vi "Start Streaming.vi"(8 "error in (no error)":errorcluster, 9 "Camera Settings":T1={"Exposure Time (ms)"=100.0, "Binning"=enum."2x2", "Scan Mode"=-1, "Frames to Acquire"=1000.0, "Pixel Correction"=FALSE, "Frames to Skip"=1, "File Path"=path "", "Duty cycle"=1.0, "ALEX"=FALSE, "Shutter Enable"=[], "fluidics trigger frame"=0, "Bit Depth"=16, "Image Width (px)"=0, "Image Height (px)"=0, "Horizontal Offset (px)"=0, "Vertical Offset (px)"=0} {"fluidics trigger frame" max=60000 step=1; "Exposure Time (ms)" min=1.0 max=10000.0 step=1.0}, 11 "Arduino In":refnum<class "Arduino DAQ.lvclass">) -> (0 "error out":errorcluster, 3 "Arduino Out":refnum<class "Arduino DAQ.lvclass">)   [LabVIEW 2023, in "Arduino DAQ.lvlib" / "Arduino DAQ.lvclass"]
uses:
  Arduino DAQ.lvclass
  Resources/Type Defs/Camera Settings.ctl
  Arduino DAQ.lvclass/Arduino DAQ.ctl
  Resources/GLOBAL/GLOBAL Time-critical.vi
  Sync Device/Sync Device.lvclass
  Arduino DAQ.lvlib
panel:
  out "shutter (us)":i32=100 min=100 max=1000000 step=1000
  out "readout (us)":i32
  out "exposure (us)":i32
  out "acquisition period (us)":i32
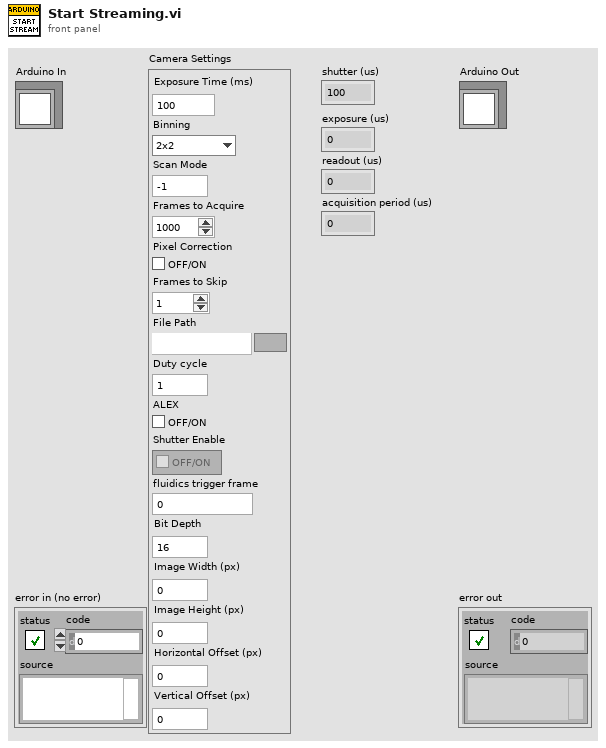
[diagram p1: front panel]
types:
  T1 = typedef "Camera Settings.ctl" = cluster{"Exposure Time (ms)":dbl, "Binning":enum16{"1x1", "2x2", "4x4"}, "Scan Mode":i32, "Frames to Acquire":dbl, "Pixel Correction":bool, "Frames to Skip":u32, "File Path":path, "Duty cycle":dbl, "ALEX":bool, "Shutter Enable":bool[], "fluidics trigger frame":u16, "Bit Depth":u16, "Image Width (px)":u16, "Image Height (px)":u16, "Horizontal Offset (px)":u16, "Vertical Offset (px)":u16}
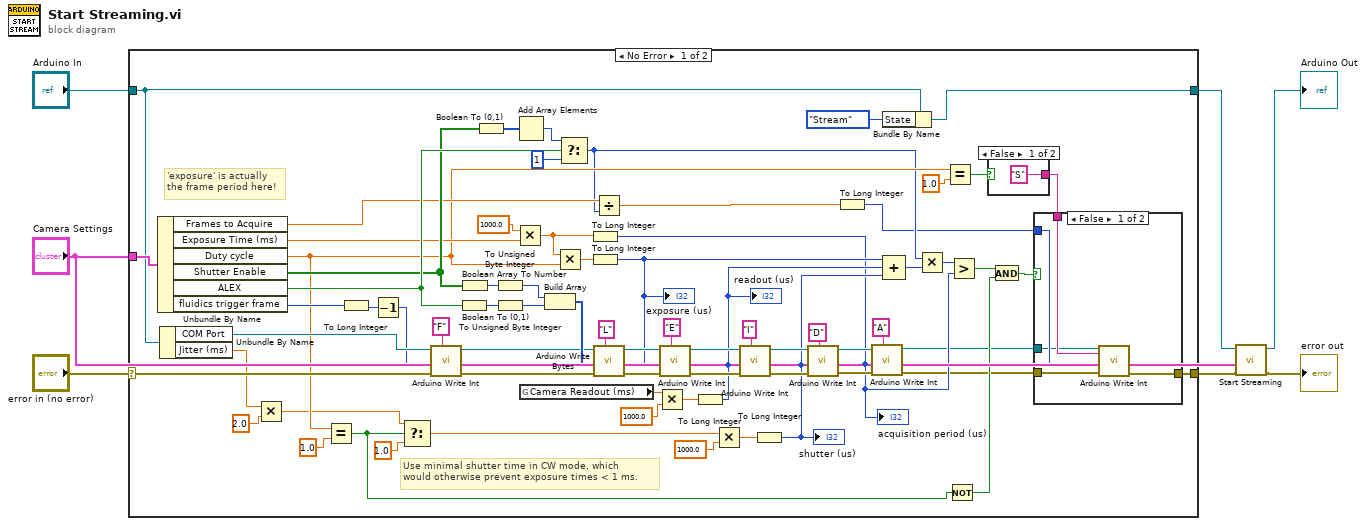
[diagram p0: block diagram]
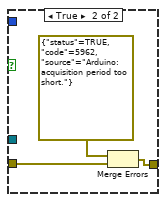
[diagram p2: hidden frame]
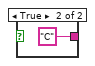
[diagram p3: hidden frame]
diagram:
  n1 = case shown="No Error" "error in (no error)" {
    selector: "error in (no error)" -> [w46 w90]
    tunnel: [w12 w90] -> w5
    tunnel: [w62 w89] -> w1
    tunnel: "Arduino In" -> [w41 w89]
    tunnel: "Camera Settings" -> [w75 _]
    frame No Error {
      # "Use minimal shutter time in CW mode, which\nwould otherwise prevent exposure times < 1 ms."
      # "'exposure' is actually\nthe frame period here!"
      n2 = Unbundle By Name(w75) -> ("Frames to Acquire"=w42:dbl, "Exposure Time (ms)"=w40:dbl, "Duty cycle"=w31:dbl, "Shutter Enable"=w57:bool[], "ALEX"=w58:bool, "fluidics trigger frame"=w36:u16)
      n3 = Unbundle By Name(w41) -> ("COM Port"=w45:refnum<visa-resource-name>, "Jitter (ms)"=w32:dbl)
      n4 = Multiply(x=w32, y=2.0) -> (x*y=w30:dbl)
      n5 = Equal?(x=w31, y=1.0) -> (x = y?=w14:bool)
      n6 = To Long Integer(number=w36) -> (32bit integer=w35:i32)
      n7 = Decrement(x=w35) -> (x-1=w34:i32)
      n8 = Select(t=w30, s=w14, f=1.0) -> (s? t:f=w28:dbl)
      n9 = call "Arduino Write Int.vi"("Command"="F", "error in (no error)"=w46, "Data"=w34, "COM Port In"=w45) -> ("error out"=w47:errorcluster, "COM Port Out"=w43:refnum<visa-resource-name>)  [unwired: 6 in]
      n10 = Boolean To (0,1)(Boolean=w58) -> (0, 1=w73:i16)
      n11 = Boolean Array To Number(Boolean array=w57) -> (number=w76:u32)
      n12 = Boolean To (0,1)(Boolean=w57) -> (0, 1=w61:i16[])
      n13 = To Unsigned Byte Integer(number=w76) -> (unsigned 8bit integer=w77:u8)
      n14 = To Unsigned Byte Integer(number=w73) -> (unsigned 8bit integer=w74:u8)
      n15 = Multiply(x=1000.0, y=w40) -> (x*y=w71:dbl)
      n16 = Add Array Elements(numeric array=w61) -> (sum=w60:i16)
      n17 = global read "GLOBAL Time-critical.vi" "Camera Readout (ms)"() -> (w24:dbl)
      n18 = Build Array(w77, w74) -> (w78:u8[])
      n19 = Multiply(x=w71, y=w31) -> (x*y=w70:dbl)
      n20 = Select(t=w60, s=w58, f=i16 1) -> (s? t:f=w20:i16)
      n21 = To Long Integer(number=w71) -> (32bit integer=w17:i32)
      "acquisition period (us)" <- w17
      n22 = To Long Integer(number=w70) -> (32bit integer=w23:i32)
      "exposure (us)" <- w23
      n23 = Divide(x=w42, y=w20) -> (x/y=w33:dbl)
      n24 = call "Arduino Write Bytes.vi"("Command"="L", "error in (no error)"=w47, "Bytes"=w78, "COM Port In"=w43) -> ("error out"=w55:errorcluster, "COM Port Out"=w56:refnum<visa-resource-name>)  [unwired: 6 in]
      n25 = Multiply(x=w24, y=1000.0) -> (x*y=w38:dbl)
      n26 = call "Arduino Write Int.vi"("Command"="E", "error in (no error)"=w55, "Data"=w23, "COM Port In"=w56) -> ("error out"=w64:errorcluster, "COM Port Out"=w65:refnum<visa-resource-name>)  [unwired: 6 in]
      n27 = To Long Integer(number=w38) -> (32bit integer=w22:i32)
      "readout (us)" <- w22
      n28 = Multiply(x=w28, y=1000.0) -> (x*y=w27:dbl)
      n29 = call "Arduino Write Int.vi"("Command"="I", "error in (no error)"=w64, "Data"=w22, "COM Port In"=w65) -> ("error out"=w67:errorcluster, "COM Port Out"=w66:refnum<visa-resource-name>)  [unwired: 6 in]
      n30 = To Long Integer(number=w27) -> (32bit integer=w21:i32)
      "shutter (us)" <- w21
      n31 = call "Arduino Write Int.vi"("Command"="D", "error in (no error)"=w67, "Data"=w21, "COM Port In"=w66) -> ("error out"=w54:errorcluster, "COM Port Out"=w48:refnum<visa-resource-name>)  [unwired: 6 in]
      n32 = To Long Integer(number=w33) -> (32bit integer=w10:i32)
      n33 = call "Arduino Write Int.vi"("Command"="A", "error in (no error)"=w54, "Data"=w17, "COM Port In"=w48) -> ("error out"=w8:errorcluster, "COM Port Out"=w9:refnum<visa-resource-name>)  [unwired: 6 in]
      n34 = Bundle By Name(cluster=w41, "State"=enum16{"Idle", "Manual", "Stream"}."Stream") -> (w62:refnum<class "Arduino DAQ.lvclass">)
      n35 = Compound Arithmetic op=ADD(w23, w22, w21) -> (w19:i32)
      n36 = Multiply(x=w20, y=w19) -> (x*y=w18:i32)
      n37 = Equal?(x=w31, y=1.0) -> (x = y?=w69:bool)
      n38 = Not(x=w14) -> (.not. x?=w13:bool)
      n39 = Greater?(x=w18, y=w17) -> (0:w16:bool)
      n40 = case shown="False" w69 {
        tunnel: ["S" ("Command") "C" ("Command")] -> w11
        frame False {
        }
        frame True {
        }
      }
      n41 = And(x=w16, y=w13) -> (x .and. y?=w15:bool)
      n42 = case shown="False" w15 {
        tunnel: [w80 w84] -> w12
        tunnel: w11 -> [w83 _]
        tunnel: w10 -> [w82 _]
        tunnel: w9 -> [w81 _]
        tunnel: w8 -> [w79 w85]
        frame False {
          n43 = call "Arduino Write Int.vi"("Command"=w83, "error in (no error)"=w79, "Data"=w82, "COM Port In"=w81) -> ("error out"=w80:errorcluster)  [unwired: 6 in, 1 out]
        }
        frame True {
          n44 = Merge Errors(errorcluster {"status"=TRUE, "code"=5962, "source"="Arduino: acquisition period too short."} ("error out"), w85) -> (w84:errorcluster)
        }
      }
    }
    frame Error {
    }
  }
  n45 = call-parent "Start Streaming.vi"("error in (no error)"=w5, "Camera Settings"="Camera Settings", "Synchronization Device in"=w1) -> ("error out"=→"error out":errorcluster, "Synchronization Device out"=→"Arduino Out":refnum<class "Arduino DAQ.lvclass">)  [unwired: 7 in]
